vi "Step Process.vi"(7 "Step State in":T1, 8 "error in (no error)":errorcluster, 9 "result allocation":T2, 10 "parameters":T2, 11 "Step in":refnum<class "Step.lvclass">) -> (0 "error out":errorcluster, 1 "results":T2, 2 "parameter allocation":T2, 3 "Step out":refnum<class "Step.lvclass">, 4 "Step State out":T1)   [LabVIEW 2015, in "Step.lvclass"]
uses:
  Step.lvclass
  <vilib>/NI/Tag Bus/table/data table.ctl
  StepState.ctl
  <vilib>/NI/Tag Bus/table/data table.lvlib
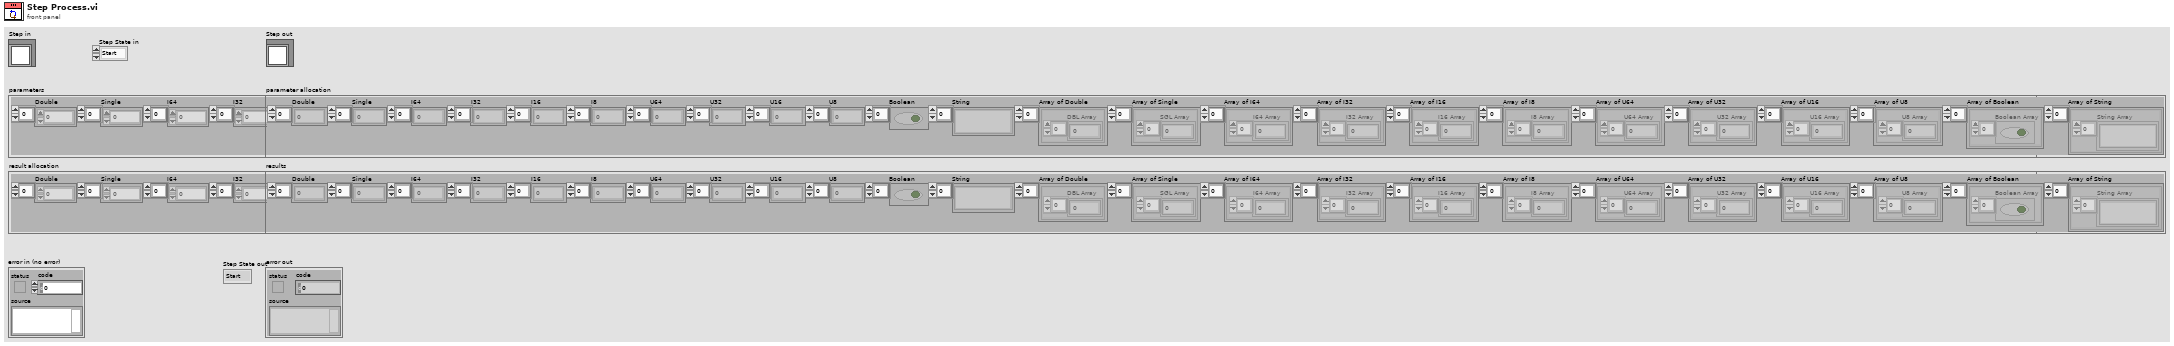
[diagram p1: front panel]
types:
  T1 = typedef "Step.lvclass/StepState.ctl" = enum16{"Start", "Skipped", "Completed", "Running", "Aborted"}
  T2 = typedef "tag bus.lvlib/data table.lvlib/data table.ctl" = cluster{"Double":dbl[], "Single":sgl[], "I64":i64[], "I32":i32[], "I16":i16[], "I8":i8[], "U64":u64[], "U32":u32[], "U16":u16[], "U8":u8[], "Boolean":bool[], "String":string[], "Array of Double":cluster{"DBL Array":dbl[]}[], "Array of Single":cluster{"SGL Array":sgl[]}[], "Array of I64":cluster{"I64 Array":i64[]}[], "Array of I32":cluster{"I32 Array":i32[]}[], "Array of I16":cluster{"I16 Array":i16[]}[], "Array of I8":cluster{"I8 Array":i8[]}[], "Array of U64":cluster{"U64 Array":u64[]}[], "Array of U32":cluster{"U32 Array":u32[]}[], "Array of U16":cluster{"U16 Array":u16[]}[], "Array of U8":cluster{"U8 Array":u8[]}[], "Array of Boolean":cluster{"Boolean Array":bool[]}[], "Array of String":cluster{"String Array":string[]}[]}
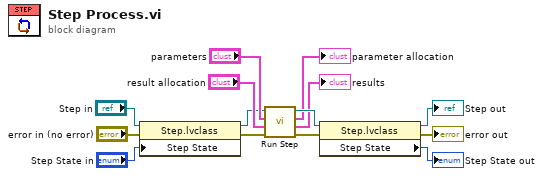
[diagram p0: block diagram]
diagram:
  n1 = property class="Step.lvclass"(reference="Step in", error in="error in (no error)", "Step State"="Step State in") -> (reference out=w11:refnum<class "Step.lvclass">, error out=w3:errorcluster)
  n2 = call-dynamic "Run Step.vi"("error in (no error)"=w3, "result allocation"="result allocation", "parameters"="parameters", "Step in"=w11) -> ("error out"=w2:errorcluster, "results"=→"results":T2, "parameter allocation"=→"parameter allocation":T2, "Step out"=w10:refnum<class "Step.lvclass">)  [unwired: 4 in]
  n3 = property class="Step.lvclass"(reference=w10, error in=w2) -> (reference out=→"Step out":refnum<class "Step.lvclass">, error out=→"error out":errorcluster, "Step State"=→"Step State out":T1)
